vi "screentest.vi"() -> ()   [LabVIEW 2014]
uses:
  <vilib>/vision/NI_Vision_Development_Module.lvlib
panel:
  in  "Boolean":bool
  in  "stop":bool
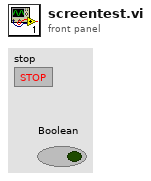
[diagram p1: front panel]
types:
  T1 = typedef "IMAQ Image.ctl" = refnum<image>
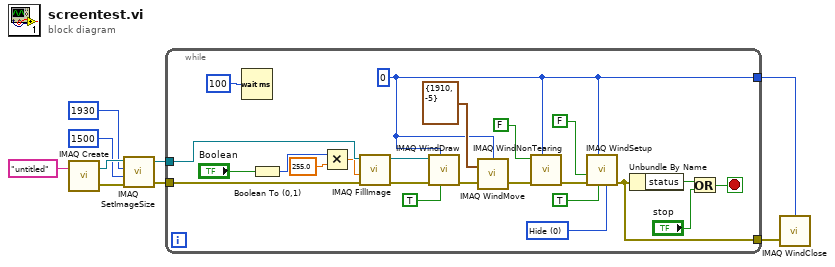
[diagram p0: block diagram]
diagram:
  n1 = call "IMAQ Create"("Image Name"="untitled") -> ("New Image"=w8:T1, "error out"=w3:errorcluster)  [unwired: 4 in]
  n2 = call "IMAQ SetImageSize"("error in (no error)"=w3, "Y Resolution"=1500 ("X Resolution"), "X Resolution"=1930, "Image"=w8) -> ("error out"=w4:errorcluster, "Image Out"=w5:T1)  [unwired: 1 in]
  n3 = while {
    tunnel: w5 -> [w27]
    tunnel: w4 -> [w20]
    tunnel: [w10] -> w2
    tunnel: [w12] -> w1
    stop <- w16 stop-if-true
    w13 = 0 items=["Hide", "Show", "No change"] ("Scrollbars (No change)")
    w12 = 0 ("Window Number (0...15)")
    n4 = Wait (ms)(milliseconds to wait=u32 100) -> ()  [unwired: 1 out]
    n5 = Boolean To (0,1)(Boolean="Boolean") -> (0, 1=w22:i16)
    n6 = Multiply(x=w22, y=255.0) -> (x*y=w21:dbl)
    n7 = call "IMAQ FillImage"("error in (no error)"=w20, "Pixel Value (U8, U16, I16, Float)"=w21, "Image"=w27) -> ("error out"=w19:errorcluster, "Image Out"=w26:T1)  [unwired: 7 in]
    n8 = call "IMAQ WindDraw"("Resize to Image Size? (Y)"=TRUE, "Window Number (0...15)"=w12, "error in (no error)"=w19, "Image"=w26) -> ("error out"=w31:errorcluster)  [unwired: 6 in, 1 out]
    n9 = call "IMAQ WindMove"("Window Number (0...15)"=w12, "Coordinates (screen)"=cluster{"X Position":i32, "Y Position":i32} {"X Position"=1910, "Y Position"=-5}, "error in (no error)"=w31) -> ("error out"=w29:errorcluster)  [unwired: 2 in, 1 out]
    n10 = call "IMAQ WindNonTearing"("Window Number"=w12, "error in (no error)"=w29, "NonTearing? (True)"=FALSE) -> ("error out"=w11:errorcluster)  [unwired: 7 in, 1 out]
    n11 = call "IMAQ WindSetup"("Scrollbars (No change)"=w13, "Window is floating? (No)"=TRUE, "Window Number (0...15)"=w12, "error in (no error)"=w11, "Window has title bar? (Yes)"=FALSE) -> ("error out"=w10:errorcluster)  [unwired: 6 in]
    n12 = Unbundle By Name(w10) -> ("status"=w17:bool)
    n13 = Or(x=w17, y="stop") -> (x .or. y?=w16:bool)
  }
  n14 = call "IMAQ WindClose"("Window Number (0...15)"=w1, "error in (no error)"=w2) -> ()  [unwired: 4 in, 1 out]
